vi "solar_write SubscribeThisUE.vi"(8 "error in (no error)":errorcluster, 10 "Publisher Target":string, 11 "solar in":refnum<class "solar.lvclass">) -> (0 "error out":errorcluster, 3 "solar out":refnum<class "solar.lvclass">)   [LabVIEW 2018, in "solar.lvclass"]
doc: "This subscribes this target's user event to receive telemetry from the destination target whenever the destination target returns telemetry. The messages returned are prefixed with the destination target's name (i.e. 'TARGET:TLM')\nNote: The destination target can be this target so the queue process can relay user event messages to its own target's user interface loop."
uses:
  solar.lvclass
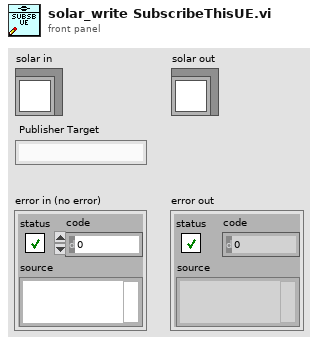
[diagram p1: front panel]
types:
  T1 = typedef "solar_ctl SOLAR Refnum.ctl" = refnum<k1>
  T2 = typedef "solar_ctl SOLAR Global.ctl" = cluster{"Targets":T3[], "AppDir":path, "solar.ini":path, "ConfigsDir":path, "CosmosDir":path, "LogsDir":path, "ExePath":path, "ExeVersion":string, "PartNum":string, "AppSetup":string, "Title":string, "Main.ini":path, "Temp.ini":path, "vSOLAR":string, "Splash.png":string, "SplashWait":i32, "SOLARUE":refnum<user-event>, "VoyagerRefnum":T4, "QTimerRefnum":T5}
  T3 = typedef "solar_ctl Target Global.ctl" = cluster{"Target":string, "Q":refnum<queue>, "UE":refnum<user-event>, "VI":refnum<vi>, "Menu":refnum<k9>, "Data":refnum<data-value>, "Attributes":variant}
  T4 = typedef "solar_voy_ctl Voyager Refnum.ctl" = refnum<k1>
  T5 = typedef "solar_qtimer_ctl Refnum.ctl" = refnum<k1>
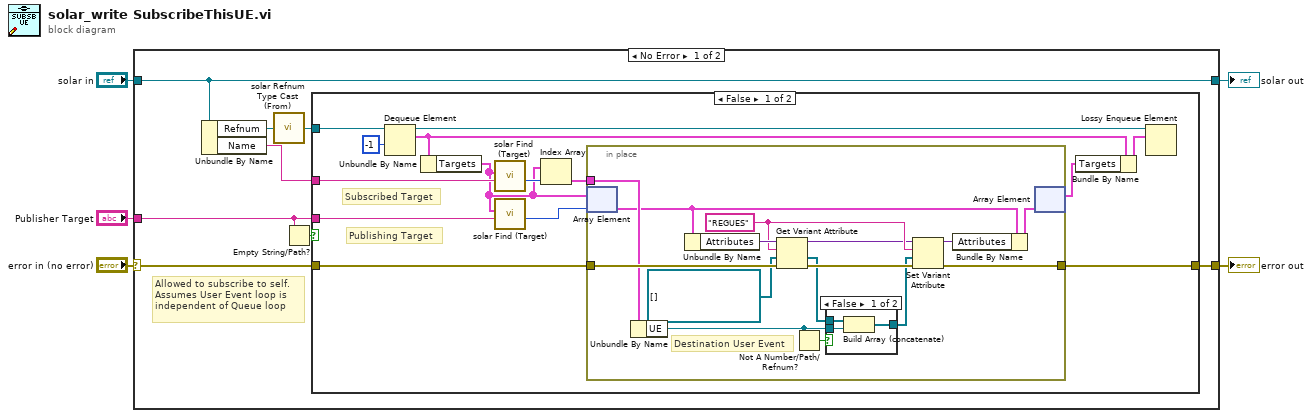
[diagram p0: block diagram]
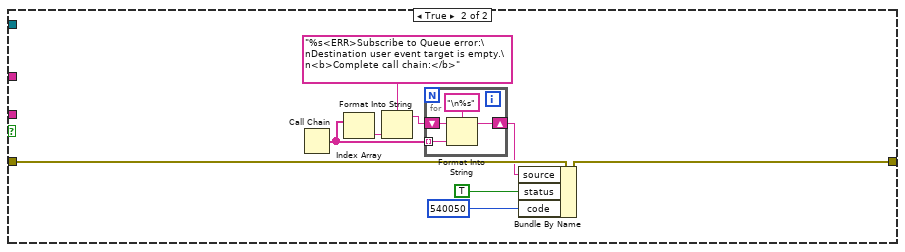
[diagram p3: hidden frame]
diagram:
  n1 = case shown="No Error" "error in (no error)" {
    selector: "error in (no error)" -> [w12 w61]
    tunnel: "solar in" -> [w13 w60]
    tunnel: [w9 w61] -> w3
    tunnel: [w13 w60] -> w1
    tunnel: "Publisher Target" -> [w7 _]
    frame No Error {
      # "Allowed to subscribe to self.\nAssumes User Event loop is\nindependent of Queue loop"
      n2 = Unbundle By Name(w13) -> ("Refnum"=w11:T1, "Name"=w8:string)
      n3 = call "solar Refnum Type Cast (From).vi"("Refnum"=w11) -> ("SOLAR"=w10:refnum<queue>)
      n4 = Empty String/Path?(string/path=w7) -> (empty?=w6:bool)
      n5 = case shown="False" w6 {
        tunnel: w12 -> [w27 w49]
        tunnel: w10 -> [w26 _]
        tunnel: [w23 w47] -> w9
        tunnel: w8 -> [w16 _]
        tunnel: w7 -> [w15 _]
        frame False {
          # "Publishing Target"
          # "Subscribed Target"
          n6 = Dequeue Element(queue=w26, timeout in ms (-1)=-1) -> (queue out=w25:refnum<queue>, element=w22:T2)  [unwired: 1 in, 2 out]
          n7 = Unbundle By Name(w22) -> ("Targets"=w14:T3[])
          n8 = call "solar Find (Target).vi"("Target"=w16, "Targets"=w14) -> ("Target Index"=w18:i32)  [unwired: 8 in, 1 out]
          n9 = call "solar Find (Target).vi"("Target"=w15, "Targets"=w14) -> ("Target Index"=w20:i32)  [unwired: 8 in, 1 out]
          n10 = Index Array(array=w14, index=w18) -> (element=w17:T3)
          n11 = in-place {
            in-place-border: w27 -> [w40]
            in-place-border: [w39] -> w23
            in-place-border: w17 -> [w29]
            w36 = "REGUES" ("name")
            # "Destination User Event"
            n12 = in-place-array #1(w14, w20) -> (w28:T3)
            n13 = Unbundle By Name(w29) -> ("UE"=w31:refnum<user-event>)
            n14 = Unbundle By Name(w28) -> ("Attributes"=w37:variant)
            n15 = Get Variant Attribute(Variant=w37, name=w36, default value (empty Variant)=refnum<user-event>[] [] ("RegUEs"), error in=w40) -> (duplicate Variant=w35:variant, value=w33:refnum<user-event>[], error out=w38:errorcluster)  [unwired: 1 out]
            n16 = Not A Number/Path/Refnum?(number/path/refnum=w31) -> (NaN/Path/Refnum?=w34:bool)
            n17 = case shown="False" w34 {
              tunnel: w33 -> [w45 w46]
              tunnel: [w44 w46] -> w32
              tunnel: w31 -> [w43 _]
              frame False {
                n18 = Build Array (concatenate)(w45, w43) -> (w44:refnum<user-event>[])
              }
              frame True {
              }
            }
            n19 = Set Variant Attribute(Variant=w35, name=w36, value=w32, error in=w38) -> (Variant out=w41:variant, error out=w39:errorcluster)  [unwired: 1 out]
            n20 = Bundle By Name(cluster=w28, "Attributes"=w41) -> (w42:T3)
            n21 = in-place-array #1(w42) -> (w19:T3[])  [unwired: 1 out]
          }
          n22 = Bundle By Name(cluster=w22, "Targets"=w19) -> (w21:T2)
          n23 = Lossy Enqueue Element(queue=w25, element=w21) -> ()  [unwired: 1 in, 4 out]
        }
        frame True {
          n24 = Call Chain() -> (call chain=w50:string[])
          n25 = Index Array(array=w50) -> (element=w52:string)  [unwired: 1 in]
          n26 = Format Into String(format string="%s<ERR>Subscribe to Queue error:\nDestination user event target is empty.\n<b>Complete call chain:</b>", w52) -> (resulting string=w51:string)  [unwired: 2 in, 1 out]
          n27 = for {
            tunnel: w50 -> [w59] mode=indexing
            shift-right: [w58] -> w48
            shift-left: w51 -> [w57]
            n28 = Format Into String(format string="\n%s", initial string=w57, w59) -> (resulting string=w58:string)  [unwired: 1 in, 1 out]
          }
          n29 = Bundle By Name(cluster=w49, "source"=w48, "status"=TRUE, "code"=540050 ("Code")) -> (w47:errorcluster)
        }
      }
    }
    frame Error {
    }
  }
  "error out" <- w3
  "solar out" <- w1
